vi "Time from Velocities and Acceleration.vi"(9 "Acceleration (in/s2)":dbl, 10 "Final Velocity (in/s)":dbl, 11 "Initial Velocity (in/s)":dbl) -> (3 "Time (s)":dbl)   [LabVIEW 2019, in "Motion Profile Generator.lvclass"]
uses:
  Motion Profile Generator.lvclass
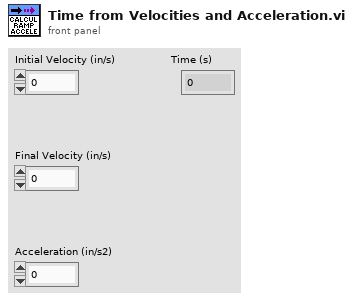
[diagram p1: front panel]
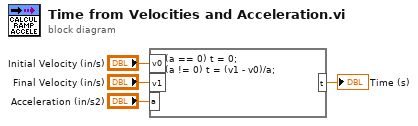
[diagram p0: block diagram]
diagram:
  n1 = formula code="if(a == 0) t = 0;\nif(a != 0) t = (v1 - v0)/a;"("v0"="Initial Velocity (in/s)", "v1"="Final Velocity (in/s)", "a"="Acceleration (in/s2)") -> ("t"=→"Time (s)":dbl)
